vi "GenNet-Client Send Notification.vi"(8 "error in":errorcluster, 10 "Original Message Data":variant, 11 "Received Message Data":variant) -> (0 "error out":errorcluster)   [LabVIEW 2014, in "GenNet-Client.lvlib"]
doc: "Sends the data that was received via network to the original requester by using the original notification"
uses:
  GenNet-Client.lvlib
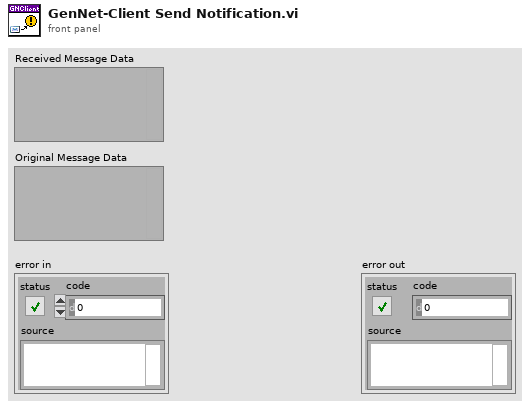
[diagram p1: front panel]
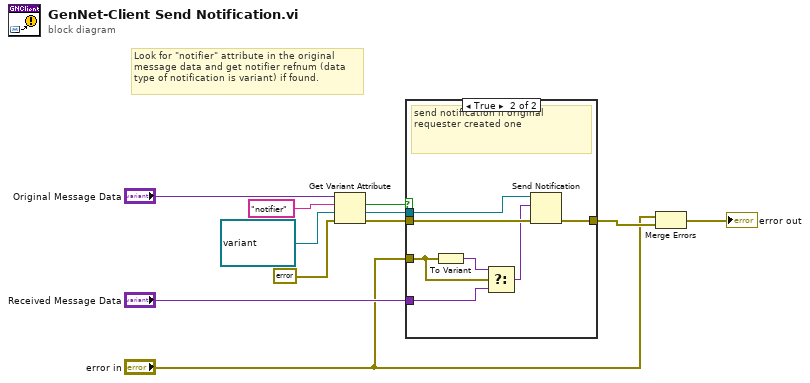
[diagram p0: block diagram]
diagram:
  # "Look for \"notifier\" attribute in the original\nmessage data and get notifier refnum (data\ntype of notification is variant) if found."
  n1 = Get Variant Attribute(Variant="Original Message Data", name="notifier", default value (empty Variant)=refnum<notifier> refnum ("notifier out"), error in=errorcluster {"status"=FALSE, "code"=0, "source"=""}) -> (found=w8:bool, value=w5:refnum<notifier>, error out=w9:errorcluster)  [unwired: 1 out]
  n2 = case shown="True" w8 {
    tunnel: w9 -> [w12 w19]
    tunnel: [w12 w18] -> w2
    tunnel: "Received Message Data" -> [_ w16]
    tunnel: w5 -> [_ w17]
    tunnel: "error in" -> [_ w15]
    frame False {
    }
    frame True {
      # "send notification if original requester created one"
      n3 = To Variant(anything=w15) -> (Variant=w13:variant)
      n4 = Select(t=w13, s=w15, f=w16) -> (s? t:f=w14:variant)
      n5 = Send Notification(notification=w14, notifier=w17, error in (no error)=w19) -> (error out=w18:errorcluster)  [unwired: 1 out]
    }
  }
  n6 = Merge Errors("error in", w2) -> (→"error out":errorcluster)
